vi "Write Formatters.vi"(8 "error in (no error)":errorcluster, 10 "Formatters":refnum<class "Formatter.lvclass">[](array[class]), 11 "ResultProcessor Config in":refnum<class "ResultProcessor Config.lvclass">) -> (0 "error out":errorcluster, 3 "ResultProcessor Config out":refnum<class "ResultProcessor Config.lvclass">)   [LabVIEW 2015, in "ResultProcessor Config.lvclass"]
uses:
  ResultProcessor Config.lvclass
  Report Formatters/Formatter.lvclass
  ResultProcessor Config.lvclass/ResultProcessor Config.ctl
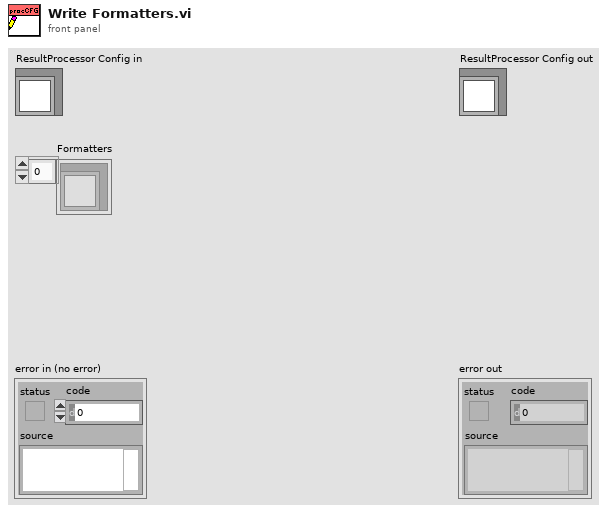
[diagram p1: front panel]
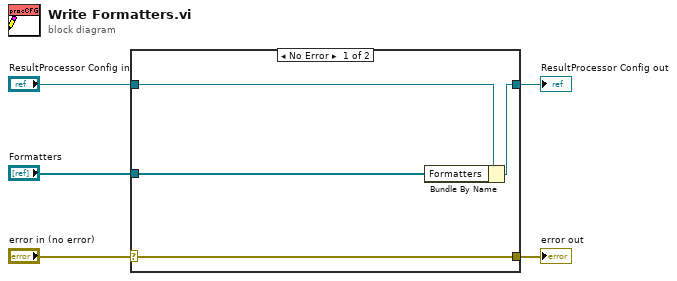
[diagram p0: block diagram]
diagram:
  n1 = case shown="No Error" "error in (no error)" {
    selector: "error in (no error)" -> [w9 w10]
    tunnel: [w9 w10] -> w4
    tunnel: [w7 w11] -> w2
    tunnel: "ResultProcessor Config in" -> [w8 w11]
    tunnel: "Formatters" -> [w6 _]
    frame No Error {
      n2 = Bundle By Name(cluster=w8, "Formatters"=w6) -> (w7:refnum<class "ResultProcessor Config.lvclass">)
    }
    frame Error {
    }
  }
  "error out" <- w4
  "ResultProcessor Config out" <- w2
